vi "Array Investigation Part 3.vi"() -> ()   [LabVIEW 2014]
doc: "This VI is an exercise in the LabVIEW Core I course.\n\nEnter the number of columns and rows you want generated, then run the VI. This VI generates an array with the number of rows and columns you specify."
panel:
  out "2nd row":dbl[](array[numeric])
  out "3rd row":dbl[](array[numeric])
  out "Intensity Graph":dbl[][](graph)
  out "Array":dbl[][](array[numeric])
  in  "Rows":i32=80
  in  "Columns":i32=80
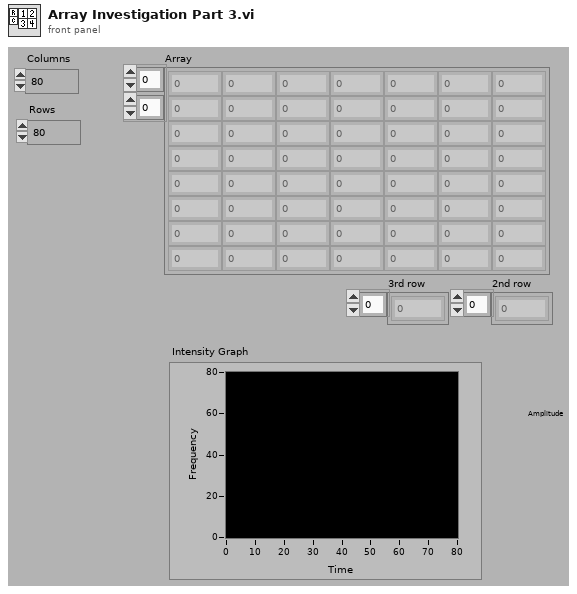
[diagram p1: front panel]
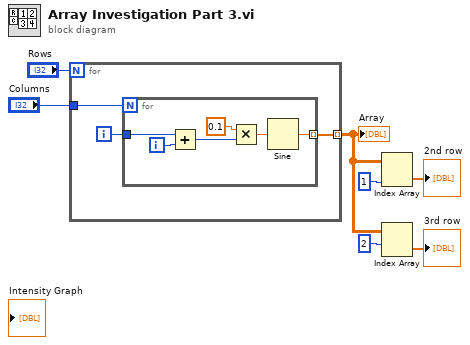
[diagram p0: block diagram]
diagram:
  n1 = for {
    N: "Rows" -> [_]
    tunnel: [w10] -> w3 mode=indexing
    tunnel: "Columns" -> [w9]
    i -> [w8]
    n2 = for {
      N: w9 -> [_]
      tunnel: [w16] -> w10 mode=indexing
      tunnel: w8 -> [w13]
      i -> [w14]
      n3 = Add(x=w13, y=w14) -> (x+y=w15:i32)
      n4 = Multiply(x=0.1, y=w15) -> (x*y=w12:dbl)
      n5 = Sine(x=w12) -> (sin(x)=w16:dbl)
    }
  }
  "Array" <- w3
  n6 = Index Array(array=w3, index (col)=1 ("disabled index (col)")) -> (element=→"2nd row":dbl[])  [unwired: 1 in]
  n7 = Index Array(array=w3, index (row)=2 ("index")) -> (element=→"3rd row":dbl[])  [unwired: 1 in]
